vi "SW_Get_1D_Array_normalize.vi"(2 "Error In":errorcluster, 4 "1D array":dbl[](array[numeric])) -> (0 "Error Out":errorcluster, 1 "Normalized 1D array":dbl[](array[numeric]))   [LabVIEW 2018, in "Tracker.lvlib"]
uses:
  Tracker.lvlib
panel:
  in  "N points":u16=300
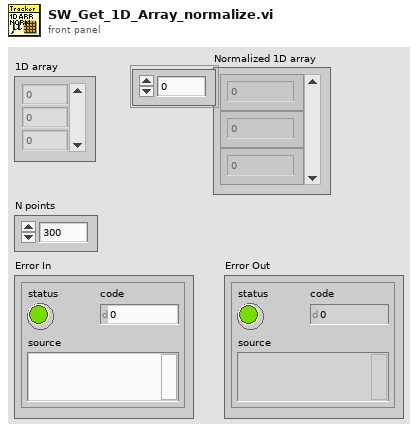
[diagram p1: front panel]
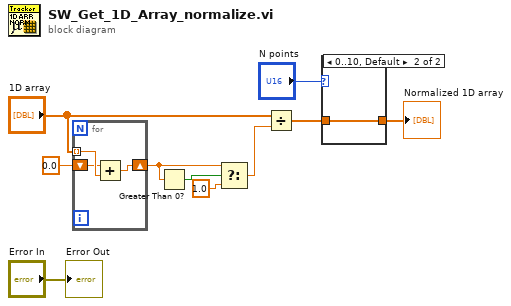
[diagram p0: block diagram]
diagram:
  n1 = for {
    tunnel: "1D array" -> [w13] mode=indexing
    shift-right: [w12] -> w3
    shift-left: 0.0 -> [w11]
    n2 = Add(x=w11, y=w13) -> (x+y=w12:dbl)
  }
  n3 = Greater Than 0?(x=w3) -> (x > 0?=w4:bool)
  n4 = Select(t=w3, s=w4, f=1.0) -> (s? t:f=w2:dbl)
  n5 = Divide(x="1D array", y=w2) -> (x/y=w6:dbl[])
  n6 = case shown="0..10, Default" "N points" {
    tunnel: [w14 w15] -> w7
    tunnel: w6 -> [w14 w15]
    frame 11.. {
    }
    frame 0..10, Default {
    }
  }
  "Normalized 1D array" <- w7
  "Error Out" <- "Error In"
